vi "DAQ_Initialization.vi"(4 "AO Lasers":tag="USB-6363/ao0:3", 5 "AO Z":tag="USB-6211/ao1", 6 "AO Pockels":tag="USB-6211/ao0", 7 "DO":tag="USB-6363/port0/line0:4", 8 "error in (no error)":errorcluster, 9 "Counter":tag="USB-6363/ctr0", 10 "Timing source":tag="OnboardClock") -> (0 "error out":errorcluster)   [LabVIEW 2025]
uses:
  <vilib>/DAQmx/create/channels.llb/DAQmx Create Channel (CO-Pulse Generation-Time).vi
  <vilib>/DAQmx/configure/events/hardwareSignals.llb/DAQmx Export Signal (Most Signals).vi
  <vilib>/DAQmx/create/channels.llb/DAQmx Create Channel (DO-Digital Output).vi
  <vilib>/DAQmx/configure/timing.llb/DAQmx Timing (Sample Clock).vi
  <vilib>/DAQmx/configure/trigger.llb/DAQmx Start Trigger (Digital Edge).vi
  <vilib>/DAQmx/create/channels.llb/DAQmx Create Channel (AO-Voltage-Basic).vi
  <resource>/objmgr/daqmx.rc
panel:
  in  "Export_Trigger":tag="/USB-6363/PFI0"
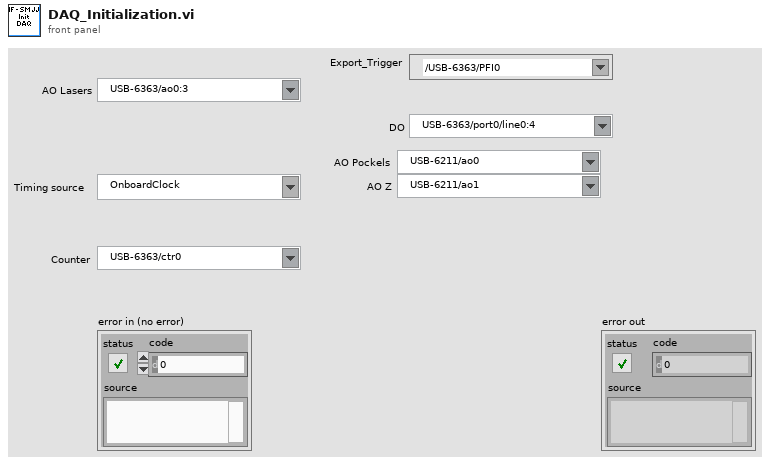
[diagram p1: front panel]
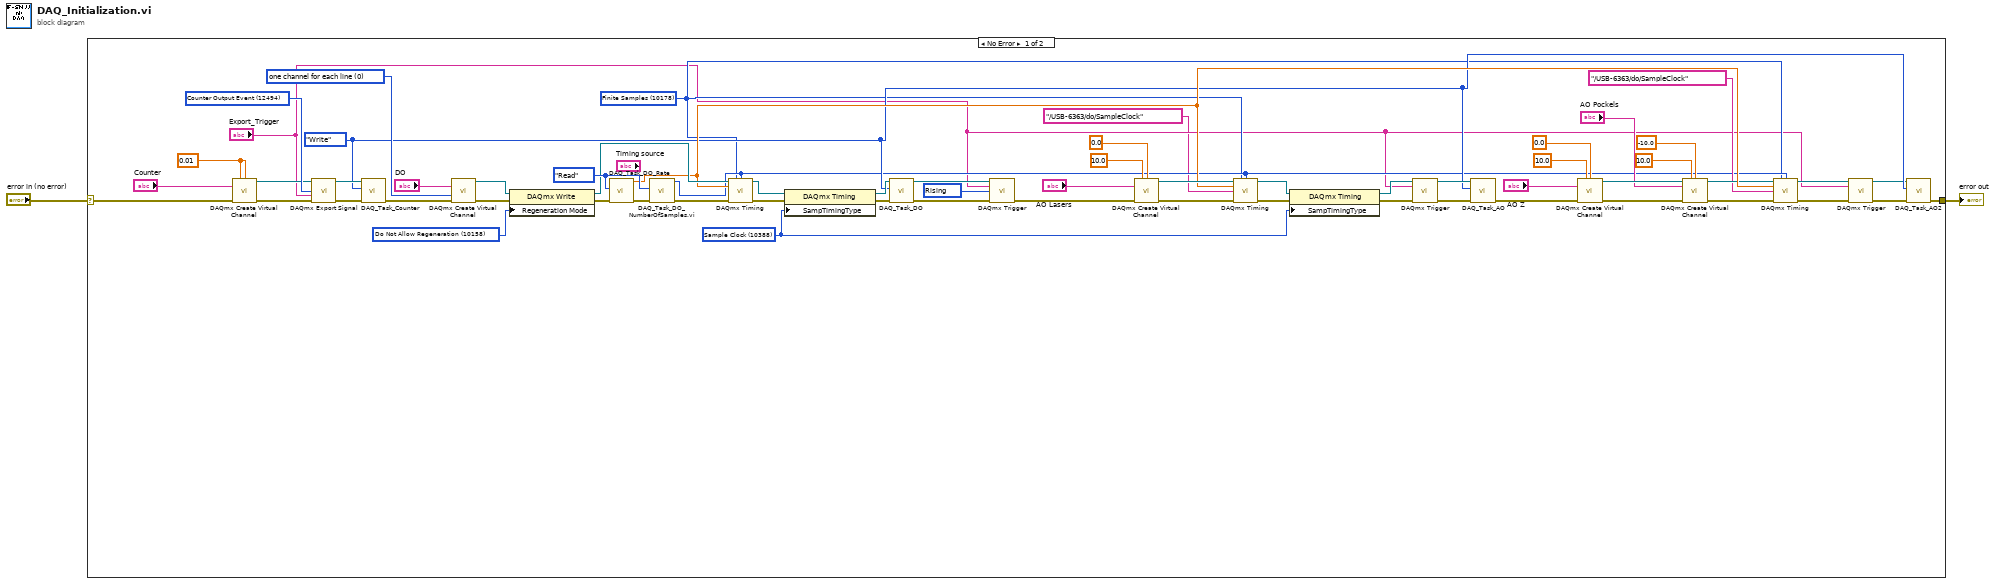
[diagram p0: block diagram]
diagram:
  n1 = case shown="No Error" "error in (no error)" {
    selector: "error in (no error)" -> [w45 w65]
    tunnel: [w19 w65] -> w1
    frame No Error {
      w31 = 12494 items=["AI Convert Clock"=12484, "10MHz Reference Clock"=12536, "20MHz Timebase Clock"=12486, "Sample Clock"=12487, "Advance Trigger"=12488, "Reference Trigger"=12490, "Start Trigger"=12491, "Advance Complete Event"=12492, "AI Hold Complete Event"=12493, "Counter Output Event"=12494, "Change Detection Event"=12511, "Watchdog Timer Expired Event"=12512] ("signal")
      w64 = 0 items=["one channel for each line", "one channel for all lines"] ("line grouping")
      w63 = enum16{"Write", "Read"}."Read" ("Action")
      w39 = 10388 items=["Sample Clock"=10388, "Burst Handshake"=12548, "Handshake"=10389, "Implicit"=10451, "On Demand"=10390, "Change Detection"=12504, "Pipelined Sample Clock"=14668] ("SampTimingType")
      w7 = 10178 items=["Finite Samples"=10178, "Continuous Samples"=10123] ("sample mode")
      w54 = 10158 items=["Allow Regeneration"=10097, "Do Not Allow Regeneration"=10158] ("RegenMode")
      w52 = 10280 items=["Rising"=10280, "Falling"=10171] ("edge")
      w51 = 0.01 ("low time")
      w21 = enum16{"Write", "Read"}."Write" ("Action")
      n2 = call-poly <vilib>:"DAQmx Create Virtual Channel.vi"("high time"=w51, "low time"=w51, "counter"="Counter", "error in"=w45) -> ("task out"=w30:refnum<k21>, "error out"=w29:errorcluster)  [unwired: 10 in]
      n3 = call-poly <vilib>:"DAQmx Export Signal.vi"("task/channels in"=w30, "signal"=w31, "output terminal"="Export_Trigger", "error in"=w29) -> ("task out"=w27:refnum<k21>, "error out"=w28:errorcluster)  [unwired: 10 in]
      n4 = call "DAQ_Task_Counter.vi"("error in"=w28, "Action"=w21, "DAQ_Task_Counter"=w27) -> ("error out"=w48:errorcluster)  [unwired: 7 in, 1 out]
      n5 = call-poly <vilib>:"DAQmx Create Virtual Channel.vi"("lines"="DO", "line grouping"=w64, "error in"=w48) -> ("task out"=w56:refnum<k21>, "error out"=w55:errorcluster)  [unwired: 11 in]
      n6 = property class="DAQmx Write"(reference=w56, error in=w55, "Regeneration Mode"=w54) -> (reference out=w53:refnum<k21>, error out=w60:errorcluster)
      n7 = call "DAQ_Task_DO_Rate.vi"("error in"=w60, "Action"=w63) -> ("error out"=w61:errorcluster, "DO_Rate"=w22:dbl)  [unwired: 8 in]
      n8 = call "DAQ_Task_DO_NumberOfSamples.vi.vi"("error in"=w61, "Action"=w63) -> ("error out"=w62:errorcluster, "Samples"=w8:u32)  [unwired: 8 in]
      n9 = call-poly <vilib>:"DAQmx Timing.vi"("task/channels in"=w53, "sample mode"=w7, "samples per channel"=w8, "rate"=w22, "error in"=w62) -> ("task out"=w5:refnum<k21>, "error out"=w58:errorcluster)  [unwired: 9 in]
      n10 = property class="DAQmx Timing"(reference=w5, error in=w58, "SampTimingType"=w39) -> (reference out=w59:refnum<k21>, error out=w57:errorcluster)
      n11 = call "DAQ_Task_DO.vi"("error in"=w57, "Action"=w21, "DAQ_Task_DO"=w59) -> ("error out"=w50:errorcluster, "DAQ_Task_DO"=w49:refnum<k21>)  [unwired: 7 in]
      n12 = call-poly <vilib>:"DAQmx Trigger.vi"("task/channels in"=w49, "source"="Export_Trigger", "edge"=w52, "error in"=w50) -> ("error out"=w18:errorcluster)  [unwired: 10 in, 1 out]
      n13 = call-poly <vilib>:"DAQmx Create Virtual Channel.vi"("maximum value"=10.0, "minimum value"=0.0, "physical channels"="AO Lasers", "error in"=w18) -> ("task out"=w41:refnum<k21>, "error out"=w40:errorcluster)  [unwired: 10 in]
      n14 = call-poly <vilib>:"DAQmx Timing.vi"("task/channels in"=w41, "sample mode"=w7, "samples per channel"=w8, "rate"=w22, "source"=tag "/USB-6363/do/SampleClock", "error in"=w40) -> ("task out"=w6:refnum<k21>, "error out"=w26:errorcluster)  [unwired: 8 in]
      n15 = property class="DAQmx Timing"(reference=w6, error in=w26, "SampTimingType"=w39) -> (reference out=w38:refnum<k21>, error out=w37:errorcluster)
      n16 = call-poly <vilib>:"DAQmx Trigger.vi"("task/channels in"=w38, "source"="Export_Trigger", "error in"=w37) -> ("task out"=w36:refnum<k21>, "error out"=w35:errorcluster)  [unwired: 11 in]
      n17 = call "DAQ_Task_AO.vi"("error in"=w35, "Action"=w21, "DAQ_Task_AO"=w36) -> ("error out"=w25:errorcluster)  [unwired: 7 in, 1 out]
      n18 = call-poly <vilib>:"DAQmx Create Virtual Channel.vi"("maximum value"=10.0, "minimum value"=0.0, "physical channels"="AO Z", "error in"=w25) -> ("task out"=w16:refnum<k21>, "error out"=w17:errorcluster)  [unwired: 10 in]
      n19 = call-poly <vilib>:"DAQmx Create Virtual Channel.vi"("task in"=w16, "maximum value"=10.0, "minimum value"=-10.0, "physical channels"="AO Pockels", "error in"=w17) -> ("task out"=w14:refnum<k21>, "error out"=w13:errorcluster)  [unwired: 9 in]
      n20 = call-poly <vilib>:"DAQmx Timing.vi"("task/channels in"=w14, "sample mode"=w7, "samples per channel"=w8, "rate"=w22, "source"=tag "/USB-6363/do/SampleClock", "error in"=w13) -> ("task out"=w23:refnum<k21>, "error out"=w24:errorcluster)  [unwired: 8 in]
      n21 = call-poly <vilib>:"DAQmx Trigger.vi"("task/channels in"=w23, "source"="Export_Trigger", "error in"=w24) -> ("task out"=w10:refnum<k21>, "error out"=w20:errorcluster)  [unwired: 11 in]
      n22 = call "DAQ_Task_AO2.vi"("error in"=w20, "Action"=w21, "DAQ_Task_AO2"=w10) -> ("error out"=w19:errorcluster)  [unwired: 7 in, 1 out]
    }
    frame Error {
    }
  }
  "error out" <- w1
